vi "WriteTest.vi"   [LabVIEW 2018]
uses:
  <vilib>/Utility/NIReport.llb/Report Type.ctl
  Init/AllPath.vi
  <vilib>/Utility/NIReport.llb/NI_report.lvclass
  <vilib>/Utility/NIReport.llb/NI_ReportGenerationCore.lvlib
types:
  T1 = typedef "NI_ReportGenerationCore.lvlib/Report Type.ctl" = enum16{"HTML", "Word", "Excel"}
  T2 = enum16{"maximized", "minimized", "normal", "no change"}
  T3 = cluster{"能量/功率":path, " 示波器":path, " 光谱仪":path, "偏振":path, "近远场":cluster{" 近场图片":path, " 远场图片":path, "发散角数据":path}, "参数":path, " 基路径":path, "文件名信息":path, "输出模板路径":path, "输出报告路径":path}
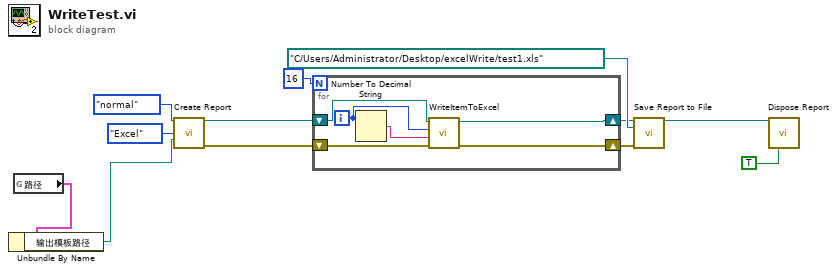
[diagram p0: block diagram]
diagram:
  n1 = global read "AllPath.vi" "路径"() -> (w2:T3)
  n2 = Unbundle By Name(w2) -> ("输出模板路径"=w1:path)
  n3 = call <vilib>:"Create Report.vi"("window state (normal)"=T2."normal", "report type"=Report_Type."Excel", "template (empty)"=w1) -> ("report out"=w7:refnum<class "NI_report.lvclass">, "error out"=w6:errorcluster)  [unwired: 11 in]
  n4 = for {
    N: 16 -> [_]
    shift-right: [w16] -> w5
    shift-left: w7 -> [w18]
    shift-right: [w15] -> w4
    shift-left: w6 -> [w17]
    i -> [w14]
    n5 = Number To Decimal String(number=w14) -> (decimal integer string=w13:string)  [unwired: 1 in]
    n6 = call "WriteItemToExcel.vi"("error in (no error)"=w17, "Data"=w13, "保存类型"=w14, "report in"=w18) -> ("error out"=w15:errorcluster, "report out"=w16:refnum<class "NI_report.lvclass">)  [unwired: 6 in]
  }
  n7 = call-dynamic "Save Report to File.vi"("report in"=w5, "report file path"=path "C:/Users/Administrator/Desktop/excelWrite/test1.xls", "error in (no error)"=w4) -> ("report out"=w10:refnum<class "NI_report.lvclass">)  [unwired: 11 in, 1 out]
  n8 = call-dynamic "Dispose Report.vi"("report in"=w10, "close report? (T)"=TRUE) -> ()  [unwired: 13 in, 1 out]
